vi "SDO_TRAJECTORY_GET_ABS_ODOM.vi"() -> (3 "Absolue Odometry":T1={"POSE"={"TRANSLATION"={"X"=0.0, "Y"=0.0}, "ROTATION"={"VALUE"=0.0, "COS"=1.0, "SIN"=0.0}}, "GyroOffset"={"VALUE"=0.0, "COS"=1.0, "SIN"=0.0}, "PreviousAngle"={"VALUE"=0.0, "COS"=1.0, "SIN"=0.0}, "PrevModulePositions"=[], "NumModules"=0} {"PrevModulePositions"."Angle"."SIN" format="%13.4f"; "PrevModulePositions"."Angle"."COS" format="%13.4f"; "PrevModulePositions"."Angle"."VALUE" format="%13.4f"; "PreviousAngle"."SIN" format="%13.4f"; "PreviousAngle"."COS" format="%13.4f"; "PreviousAngle"."VALUE" format="%13.4f"; "GyroOffset"."SIN" format="%13.4f"; "GyroOffset"."COS" format="%13.4f"; "GyroOffset"."VALUE" format="%13.4f"; "POSE"."ROTATION"."SIN" format="%13.4f"; "POSE"."ROTATION"."COS" format="%13.4f"; "POSE"."ROTATION"."VALUE" format="%13.4f"; "POSE"."TRANSLATION"."Y" format="%14.3f"; "POSE"."TRANSLATION"."X" format="%14.3f"})   [LabVIEW 2019]
uses:
  <vilib>/Rock Robotics/WPI/ThirdParty/JAS_Junk/TrajLib/TypeDef/SWERVE_DRIVE_ODOMETRY.ctl
  <vilib>/Rock Robotics/WPI/ThirdParty/JAS_Junk/TrajLib/TypeDef/POSE2D.ctl
  <vilib>/Rock Robotics/WPI/ThirdParty/JAS_Junk/TrajLib/TypeDef/TRANSLATION2D.ctl
  <vilib>/Rock Robotics/WPI/ThirdParty/JAS_Junk/TrajLib/TypeDef/ROTATION2D.ctl
  <vilib>/Rock Robotics/WPI/ThirdParty/JAS_Junk/TrajLib/TypeDef/SWERVE_DRIVE_MODULE_POSITION.ctl
  SDO_TRAJECTORY_GLOBALS.vi
  <vilib>/Rock Robotics/WPI/ThirdParty/JAS_Junk/TrajLib/Trajectory_Library.lvlib
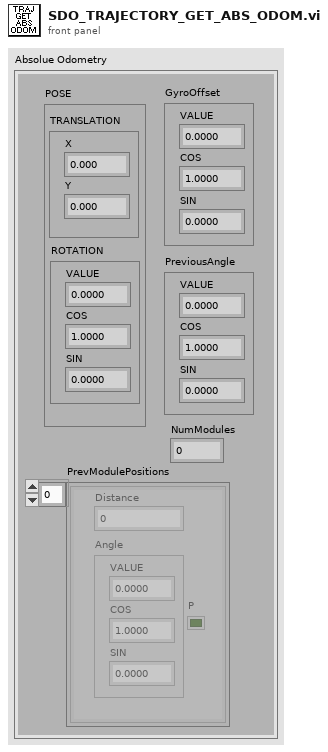
[diagram p1: front panel]
types:
  T1 = typedef "Trajectory_Library.lvlib/SWERVE_DRIVE_ODOMETRY.ctl" = cluster{"POSE":T2, "GyroOffset":T4, "PreviousAngle":T4, "PrevModulePositions":T5[], "NumModules":i32}
  T2 = typedef "Trajectory_Library.lvlib/POSE2D.ctl" = cluster{"TRANSLATION":T3, "ROTATION":T4}
  T3 = typedef "Trajectory_Library.lvlib/TRANSLATION2D.ctl" = cluster{"X":dbl, "Y":dbl}
  T4 = typedef "Trajectory_Library.lvlib/ROTATION2D.ctl" = cluster{"VALUE":dbl, "COS":dbl, "SIN":dbl}
  T5 = typedef "Trajectory_Library.lvlib/SWERVE_DRIVE_MODULE_POSITION.ctl" = cluster{"Distance":dbl, "Angle":T4, "P":bool}
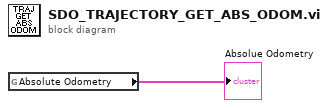
[diagram p0: block diagram]
diagram:
  n1 = global read "SDO_TRAJECTORY_GLOBALS.vi" "Absolute Odometry"() -> (→"Absolue Odometry":T1)
